vi "Network Adapter Monitor.vi"   [LabVIEW 2021]
doc: "This VI collects the netowrk adapter metadata and returns it tot he telemetry handler. The loop in this VI executes every 5 seconds."
uses:
  <vilib>/Platform/TimedLoop/XDataNode/timing_clust.ctl
  <vilib>/Platform/TimedLoop/XDataNode/nitl_modes.ctl
  <vilib>/Platform/TimedLoop/XDataNode/wakeup.ctl
  Type Definitions/Network Adapter State.ctl
  Type Definitions/Payload Class.ctl
  Type Definitions/Enum - System State.ctl
  <vilib>/platform/TimedLoop/XDataNode/XDataNode.xnode
  <vilib>/Platform/TimedLoop/XDataNode/XDNodeRunTimeDep.lvlib
types:
  T1 = typedef "XDNodeRunTimeDep.lvlib/timing_clust.ctl" = cluster{"Expected End [f-1]":u64, "Actual End [f-1]":u64, "Finished Late? [f-1]":bool, "Expected End [i-1]":u64, "Actual End [i-1]":u64, "Finished Late? [i-1]":bool, "Expected Start [i]":u64, "Actual Start [i]":u64, "Expected Start [f]":u64, "Actual Start [f]":u64, "Source Name":string, "Structure Name":string, "Period":i64, "Deadline":i64, "Offset":i64, "Start":i64, "Priority":i32, "Timeout":i32, "Mode":T2, "Wakeup Reason":T3, "Error":errorcluster, "Source Type":string, "Secondary Source Type":string, "Global End Time":u64, "Global Start Time":u64, "Frame Duration":u64, "Iteration Duration":u64, "Assigned CPU":i32, "I/O Scan Engine Mode":u32}
  T2 = typedef "XDNodeRunTimeDep.lvlib/nitl_modes.ctl" = enum32{"No Change", "Process missed periods, maintain original phase", "Discard missed periods, maintain original phase", "Process missed periods, ignore original phase", "Discard missed periods, ignore original phase"}
  T3 = typedef "XDNodeRunTimeDep.lvlib/wakeup.ctl" = enum32{"Normal", "Aborted", "Asynchronous wakeup", "Timing source error", "Timed loop error", "Timeout"}
  T4 = typedef "Enum - System State.ctl" = enum16{"System Time", "Telemetry TCP State", "Writeable Drive State", "Command TCP State", "Network Adapter State", "Discovery Engine State", "Disk State"}
  T5 = typedef "Payload Class.ctl" = enum16{"System State", "Parameters", "Metadata", "Software Monitor", "Data", "Commands"}
  T6 = typedef "Network Adapter State.ctl" = cluster{"Adapter IP Addresses":string[]}
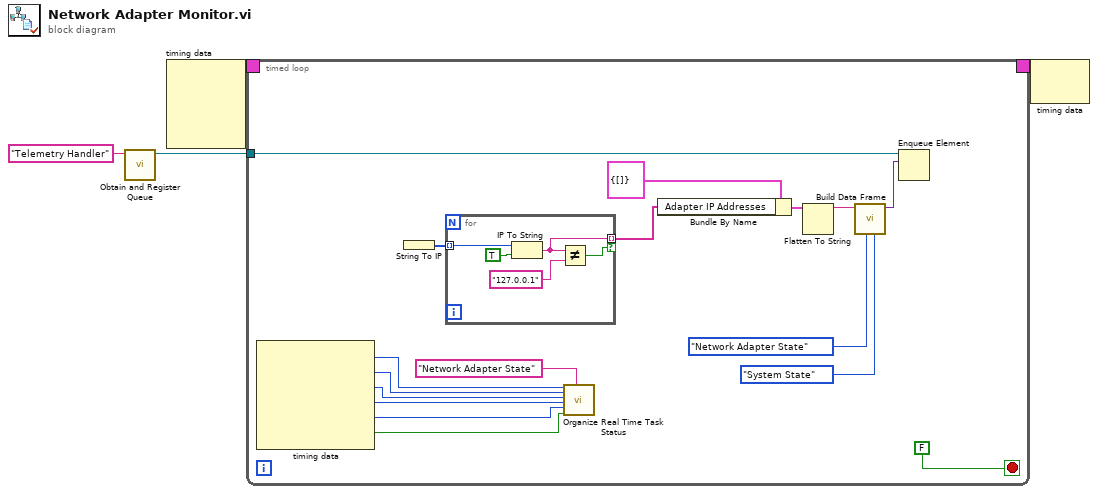
[diagram p0: block diagram]
diagram:
  n1 = call "Obtain and Register Queue.vi"("Queue Name (unnamed)"="Telemetry Handler" ("name (unnamed)")) -> ("Queue Reference"=w1:refnum<queue>)  [unwired: 9 in, 1 out]
  n2 = node-c288() -> (w4:T1)  [unwired: 4 in]
  n3 = timed-loop {
    timing: w4 -> [_]
    timing-out: [_] -> w3
    tunnel: w1 -> [w5]
    stop <- FALSE stop-if-true
    n4 = node-c288() -> (w19:i32, w18:i32, w17:i64, w16:i64, w15:i64, w14:bool)  [unwired: 1 in]
    n5 = String To IP() -> (0:w13:u32[])  [unwired: 1 in]
    n6 = for {
      tunnel: w13 -> [w26] mode=indexing
      tunnel: [w24] -> w11 mode=indexing if=w22
      n7 = IP To String(1:TRUE ("dot notation? (F)"), 2:w26) -> (0:w24:string)
      n8 = Not Equal?(x=w24, y="127.0.0.1") -> (x != y?=w22:bool)
    }
    n9 = call "Organize Real Time Task Status.vi"("Priority"=w19, "Processor"=w18, "Offset"=w17, "Iteration Duration"=w16, "Period"=w15, "Finished Late? [i-1]"=w14, "Task Name"="Network Adapter State") -> ()  [unwired: 12 in, 1 out]
    n10 = Bundle By Name(cluster=T6 {"Adapter IP Addresses"=[]}, "Adapter IP Addresses"=w11) -> (w8:T6)
    n11 = Flatten To String(anything=w8) -> (data string=w10:string)  [unwired: 3 in, 2 out]
    n12 = call "Build Data Frame.vi"("Payload Class (Data)"=Payload_Class."System State", "Payload ID (0)"=Enum_-_System_State."Network Adapter State" ("System State"), "Payload (Empty String)"=w10) -> ("Frame"=w6:variant)  [unwired: 7 in, 1 out]
    n13 = Enqueue Element(queue=w5, element=w6) -> ()  [unwired: 2 in, 3 out]
  }
  n14 = node-c288(w3) -> ()  [unwired: 1 out]
